vi "TestACS712.vi"() -> ()   [LabVIEW 2023]
panel:
  out "Waveform Graph":dynamicdata(graph)
  out "Waveform Chart":dynamicdata(graph)
  in  "?":bool
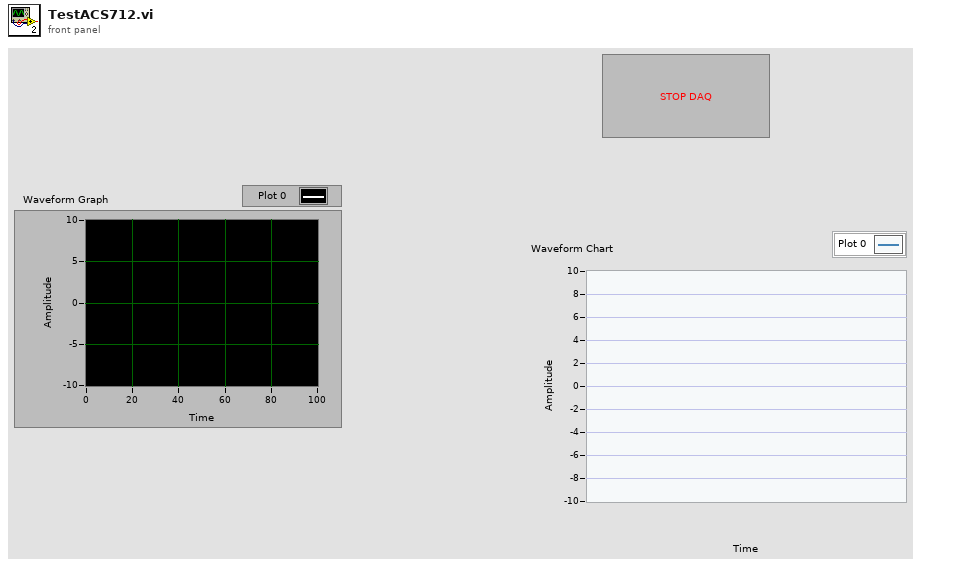
[diagram p1: front panel]
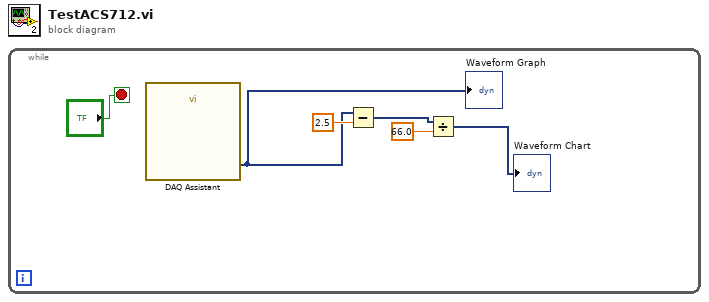
[diagram p0: block diagram]
diagram:
  n1 = while {
    stop <- "?" stop-if-true
    n2 = call "DAQ Assistant"() -> ("data"=w1:dynamicdata)  [unwired: 16 in, 3 out]
    "Waveform Graph" <- w1
    n3 = Subtract(x=w1, y=2.5) -> (x-y=w4:dynamicdata)
    n4 = Divide(x=w4, y=66.0) -> (x/y=→"Waveform Chart":dynamicdata)
  }
